vi "Test Motor Controller.vi"() -> ()   [LabVIEW 2026]
uses:
  Motor/Motor Messages/Set Speed Msg/Set Speed Msg.lvclass/Set Speed Msg.ctl
  <vilib>/ActorFramework/Message Enqueuer/Message Enqueuer.lvclass/Message Enqueuer.ctl
  <vilib>/ActorFramework/Message Enqueuer/Enqueue.vi
  Motor/Motor/Motor.lvclass
  usr/local/natinst/LabVIEW-2026-64/vi.lib/ActorFramework/Actor/Actor.lvclass
  Motor/Motor Messages/Set Speed Msg/Set Speed Msg.lvclass
  usr/local/natinst/LabVIEW-2026-64/vi.lib/ActorFramework/Message/Message.lvclass
  <vilib>/ActorFramework/Stop Msg/Stop Msg.lvclass
  <vilib>/ActorFramework/Message Priority Queue/Priority Enqueue.vi
  <vilib>/ActorFramework/Actor/Actor.lvclass
  CTI-Grove/Examples/Sourcecode/cti-drivers-lv-visa-simple/Examples/Driver/CTIPicoVISA.lvlib
panel:
  out "error out":errorcluster
  in  "stop":bool
  in  "Speed":sgl(slide) scale=-1.0..1.0
  in  "Negative Pole":i32[](array[numeric])=[7, 9, 19, 21]
  in  "Positive Pole":i32[](array[numeric])=[6, 8, 18, 20]
  in  "VISA resource name":refnum<visa-resource-name>
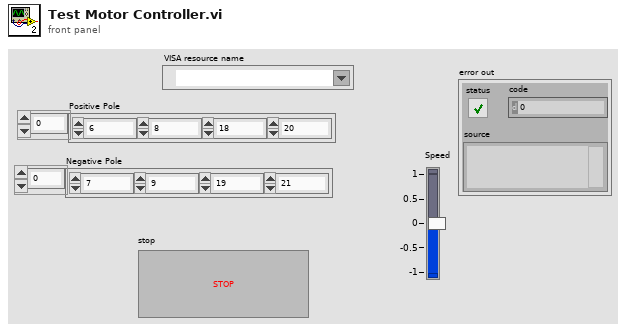
[diagram p1: front panel]
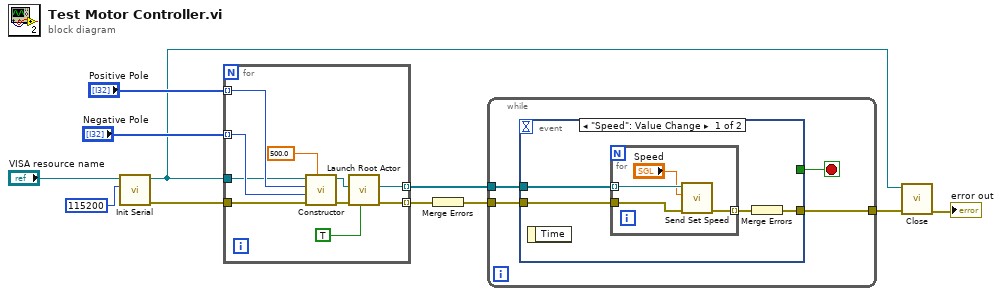
[diagram p0: block diagram]
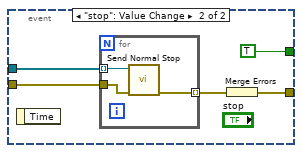
[diagram p2: hidden frame]
diagram:
  n1 = call "Init Serial.vi"("Baud (115200)"=u32 115200, "VISA resource name in"="VISA resource name") -> ("error out"=w6:errorcluster, "VISA resource name Out"=w1:refnum<visa-resource-name>)  [unwired: 7 in, 1 out]
  n2 = for {
    tunnel: "Positive Pole" -> [w21] mode=indexing
    tunnel: "Negative Pole" -> [w20] mode=indexing
    tunnel: [w16] -> w9 mode=indexing
    tunnel: w1 -> [w15]
    tunnel: w6 -> [w14]
    tunnel: [w13] -> w5 mode=indexing
    n3 = call "Constructor.vi"("Frequency"=500.0, "error in (no error)"=w14, "Negative Pole"=w20, "Positive Pole"=w21, "VISA resource name"=w15) -> ("error out"=w17:errorcluster, "Motor out"=w18:refnum<class "Motor.lvclass">)  [unwired: 5 in]
    n4 = call <vilib>:"Launch Root Actor.vi"("Open Actor Core front panel? (F)"=TRUE, "error in (no error)"=w17, "Actor"=w18) -> ("error out"=w13:errorcluster, "Actor's Enqueuer"=w16:refnum<class "Message Enqueuer.lvclass">)  [unwired: 7 in]
  }
  n5 = Merge Errors(w5) -> (w4:errorcluster)
  n6 = while {
    tunnel: w9 -> [w25]
    tunnel: [w23] -> w3
    tunnel: w4 -> [w22]
    stop <- w24 stop-if-true
    n7 = event shown="[0] \"Speed\": Value Change" {
      selector: _ -> [_ _]
      dyn-events: _ -> [_ _]
      timeout: _ -> [_ _]
      tunnel: w25 -> [w29 w38]
      tunnel: [w27 w35] -> w23
      tunnel: [_ TRUE] -> w24
      tunnel: w22 -> [w26 w34]
      event "Speed": Value Change {
        n8 = event-data() -> ()  [unwired: 1 in, 1 out]
        n9 = for {
          tunnel: w29 -> [w33] mode=indexing
          tunnel: [w31] -> w28 mode=indexing
          tunnel: w26 -> [w30]
          n10 = call "Send Set Speed.vi"("error in (no error)"=w30, "Speed"="Speed", "Message Enqueuer"=w33) -> ("error out"=w31:errorcluster)  [unwired: 7 in, 1 out]
        }
        n11 = Merge Errors(w28) -> (w27:errorcluster)
      }
      event "stop": Value Change {
        n12 = event-data() -> ()  [unwired: 1 in, 1 out]
        n13 = for {
          tunnel: w38 -> [w41] mode=indexing
          tunnel: [w40] -> w37 mode=indexing
          tunnel: w34 -> [w39]
          n14 = call <vilib>:"Send Normal Stop.vi"("error in (no error)"=w39, "Message Enqueuer"=w41) -> ("error out"=w40:errorcluster)  [unwired: 9 in]
        }
        n15 = Merge Errors(w37) -> (w35:errorcluster)
      }
    }
  }
  n16 = call "Close.vi"("error in (no error)"=w3, "VISA resource name in"=w1) -> ("error out"=→"error out":errorcluster)  [unwired: 9 in]
